vi "Get Integer Value.vi"(6 "Default Value":u32, 8 "error in (no error)":errorcluster, 10 "Name":string, 11 "Test Recipe in":refnum<class "Test Recipe.lvclass">) -> (0 "error out":errorcluster, 2 "Value":u32, 3 "Test Recipe out":refnum<class "Test Recipe.lvclass">)   [LabVIEW 2015]
uses:
  Test Recipe.lvclass
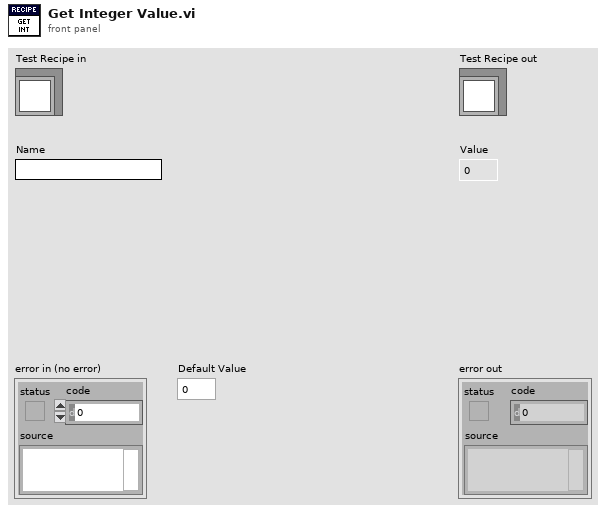
[diagram p1: front panel]
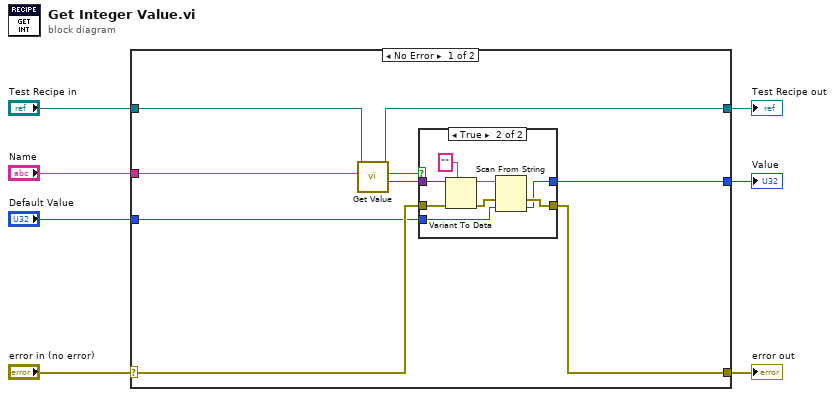
[diagram p0: block diagram]
diagram:
  n1 = case shown="No Error" "error in (no error)" {
    selector: "error in (no error)" -> [w12 w28]
    tunnel: [w9 w28] -> w6
    tunnel: [w15 w27] -> w4
    tunnel: "Test Recipe in" -> [w16 w27]
    tunnel: "Name" -> [w14 _]
    tunnel: [w10 _] -> w2
    tunnel: "Default Value" -> [w11 _]
    frame No Error {
      n2 = call-dynamic "Get Value.vi"("Key"=w14, "Registry in"=w16) -> ("Value"=w13:variant, "found?"=w8:bool, "Registry out"=w15:refnum<class "Test Recipe.lvclass">)  [unwired: 6 in, 1 out]
      n3 = case shown="True" w8 {
        tunnel: w13 -> [_ w26]
        tunnel: [w17 w20] -> w10
        tunnel: w12 -> [w18 w25]
        tunnel: [w18 w21] -> w9
        tunnel: w11 -> [w17 w19]
        frame False {
        }
        frame True {
          n4 = Variant To Data(error in=w25, type="", Variant=w26) -> (data=w23:string, error out=w22:errorcluster)
          n5 = Scan From String(input string=w23, error in=w22, default 1=w19) -> (error out=w21:errorcluster, output 1=w20:u32)  [unwired: 2 in, 2 out]
        }
      }
    }
    frame Error {
    }
  }
  "error out" <- w6
  "Test Recipe out" <- w4
  "Value" <- w2
